vi "Initialize.vi"(8 "Error In":errorcluster, 11 "lv-libssh2 Shared Library":path=path "") -> (0 "Error Out":errorcluster, 3 "SSH":refnum<class "SSH.lvclass">)   [LabVIEW 2018, in "Toolkit.lvlib" / "SSH.lvclass"]
uses:
  SSH.lvclass
  SSH.lvclass/SSH.ctl
  Toolkit.lvlib
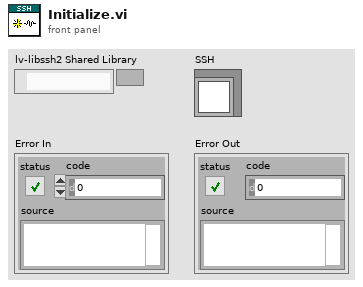
[diagram p1: front panel]
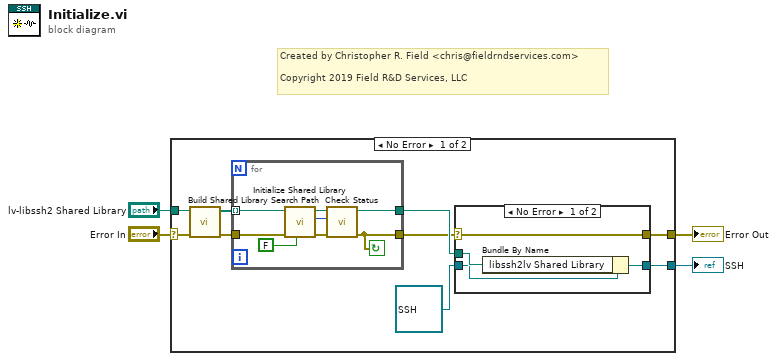
[diagram p0: block diagram]
diagram:
  # "Created by Christopher R. Field <chris@fieldrndservices.com>\n\nCopyright 2019 Field R&D Services, LLC"
  n1 = case shown="No Error" "Error In" {
    selector: "Error In" -> [w13 w28]
    tunnel: "lv-libssh2 Shared Library" -> [w12 _]
    tunnel: [w6 w28] -> w2
    tunnel: [w8 _] -> w1
    frame No Error {
      n2 = call "Build Shared Library Search Path.vi"("Error In"=w13, "libssh2lv Shared Library"=w12) -> ("Error Out"=w10:errorcluster, "Search Path"=w11:path[])  [unwired: 8 in]
      n3 = for {
        tunnel: w11 -> [w26] mode=indexing
        tunnel: w10 -> [w27]
        tunnel: [w24] -> w9
        tunnel: [w21] -> w7
        stop <- w21 continue-if-true
        n4 = call "Initialize Shared Library.vi"("Unload"=FALSE, "Error In"=w27, "libssh2lv Shared Library In"=w26) -> ("Error Out"=w22:errorcluster, "Return Code"=w23:i32, "libssh2lv Shared Library Out"=w25:path)  [unwired: 6 in]
        n5 = call "Check Status.vi"("Error In"=w22, "Status"=w23, "lv-libssh2 Shared Library In"=w25) -> ("Error Out"=w21:errorcluster, "lv-libssh2 Shared Library Out"=w24:path)  [unwired: 7 in]
      }
      n6 = case shown="No Error" w7 {
        selector: w7 -> [w15 w19]
        tunnel: w9 -> [w17 _]
        tunnel: [w16 w18] -> w8
        tunnel: [w15 w19] -> w6
        tunnel: refnum<class "SSH.lvclass"> refnum ("Toolkit.lvlib:SSH.lvclass") -> [w14 w18]
        frame No Error {
          n7 = Bundle By Name(cluster=w14, "libssh2lv Shared Library"=w17) -> (w16:refnum<class "SSH.lvclass">)
        }
        frame Error {
        }
      }
    }
    frame Error {
    }
  }
  "Error Out" <- w2
  "SSH" <- w1
